vi "DriveDistance.vi"(7 "Setpoint":dbl, 8 "error in (no error)":errorcluster, 9 "Distance":dbl, 10 "SonarMB1010AnalogDevRef":T1 {"Average Bits" max=15}, 11 "Setpoint 2":dbl) -> (0 "error out":errorcluster, 3 "Boolean":bool)   [LabVIEW 2016]
uses:
  <vilib>/Rock Robotics/WPI/Ultrasonic/WPI_SonarMB1010AnalogDeviceRef.ctl
  <vilib>/Rock Robotics/WPI/AnalogChannel/WPI_AnalogChannelDevRef.ctl
  <vilib>/Rock Robotics/SystemInterfaces/AI/FPGA_AIChannel.ctl
  <vilib>/Rock Robotics/WPI/Ultrasonic/WPI_SonarMB1010AnalogGetRange.vi
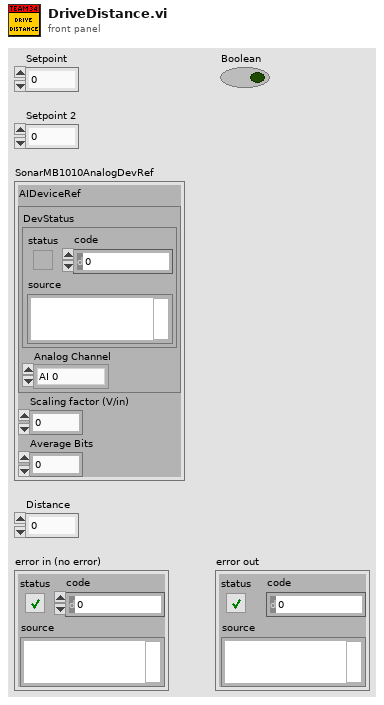
[diagram p1: front panel]
types:
  T1 = typedef "WPI_SonarMB1010AnalogDeviceRef.ctl" = cluster{"AIDeviceRef":T2, "Scaling factor (V/in)":dbl, "Average Bits":u8}
  T2 = typedef "WPI_AnalogChannelDevRef.ctl" = cluster{"DevStatus":errorcluster, "Analog Channel":T3}
  T3 = typedef "FPGA_AIChannel.ctl" = enum8{"AI 0", "AI 1", "AI 2", "AI 3", "AI MXP 0", "AI MXP 1", "AI MXP 2", "AI MXP 3", "Invalid"}
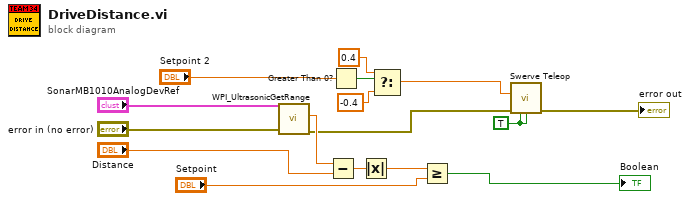
[diagram p0: block diagram]
diagram:
  w12 = TRUE ("Robot Centric?")
  n1 = call-poly <vilib>:"WPI_UltrasonicGetRange.vi"("error in"="error in (no error)", "SonarMB1010AnalogDevRef"="SonarMB1010AnalogDevRef") -> ("error out"=w6:errorcluster, "Distance"=w13:dbl)  [unwired: 7 in, 1 out]
  n2 = Subtract(x=w13, y="Distance") -> (x-y=w16:dbl)
  n3 = Greater Than 0?(x="Setpoint 2") -> (x > 0?=w11:bool)
  n4 = Absolute Value(x=w16) -> (abs(x)=w1:dbl)
  n5 = Select(t=0.4 ("Y"), s=w11, f=-0.4 ("Y")) -> (s? t:f=w8:dbl)
  n6 = Greater Or Equal?(x=w1, y="Setpoint") -> (x >= y?=→"Boolean":bool)
  n7 = call "Swerve Teleop.vi"("Y"=w8, "Error In"=w6, "Robot Centric?"=w12, "Autonomous?"=w12) -> ("Error Out"=→"error out":errorcluster)  [unwired: 7 in, 4 out]
